vi "Comparator2.vi"(0 "7-have":i32, 1 "5-code":i32, 2 "6-have":i32, 3 "6-code":i32, 4 "5- have":i32, 5 "7-code":i32, 6 "8-code":i32, 8 "4-code":i32, 9 "1-have":i32, 10 "8-have":i32, 11 "2-have":i32, 12 "3 - code":i32, 13 "3- have":i32, 14 "2-code":i32, 15 "4-have":i32, 16 "1 - code":i32) -> (18 "Enough Marbles?":bool)   [LabVIEW 2016]
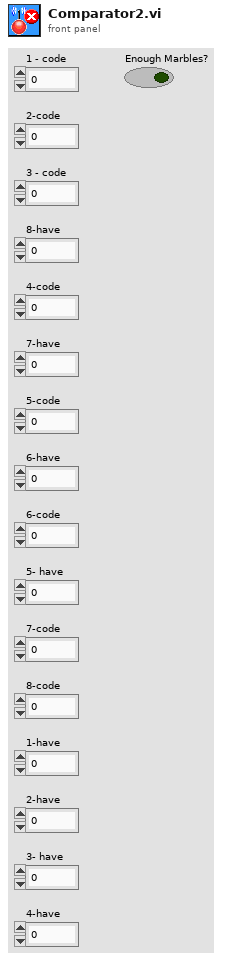
[diagram p1: front panel]
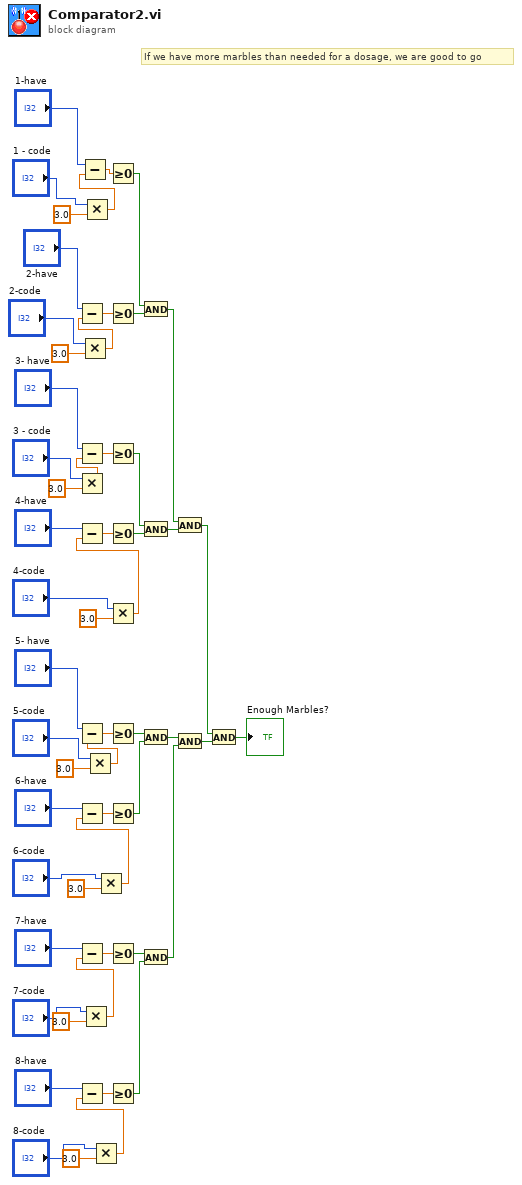
[diagram p0: block diagram]
diagram:
  # "If we have more marbles than needed for a dosage, we are good to go"
  n1 = Multiply(x="3 - code", y=3.0) -> (x*y=w17:dbl)
  n2 = Subtract(x="3- have", y=w17) -> (x-y=w35:dbl)
  n3 = Multiply(x="2-code", y=3.0) -> (x*y=w20:dbl)
  n4 = Subtract(x="2-have", y=w20) -> (x-y=w34:dbl)
  n5 = Multiply(x="7-code", y=3.0) -> (x*y=w4:dbl)
  n6 = Subtract(x="7-have", y=w4) -> (x-y=w39:dbl)
  n7 = Multiply(x="1 - code", y=3.0) -> (x*y=w23:dbl)
  n8 = Subtract(x="1-have", y=w23) -> (x-y=w33:dbl)
  n9 = Multiply(x="5-code", y=3.0) -> (x*y=w10:dbl)
  n10 = Subtract(x="5- have", y=w10) -> (x-y=w37:dbl)
  n11 = Multiply(x="8-code", y=3.0) -> (x*y=w1:dbl)
  n12 = Subtract(x="8-have", y=w1) -> (x-y=w40:dbl)
  n13 = Multiply(x="6-code", y=3.0) -> (x*y=w8:dbl)
  n14 = Subtract(x="6-have", y=w8) -> (x-y=w38:dbl)
  n15 = Greater Or Equal To 0?(x=w33) -> (x >= 0?=w41:bool)
  n16 = Greater Or Equal To 0?(x=w34) -> (x >= 0?=w42:bool)
  n17 = Greater Or Equal To 0?(x=w35) -> (x >= 0?=w43:bool)
  n18 = Multiply(x="4-code", y=3.0) -> (x*y=w13:dbl)
  n19 = Subtract(x="4-have", y=w13) -> (x-y=w36:dbl)
  n20 = Greater Or Equal To 0?(x=w36) -> (x >= 0?=w44:bool)
  n21 = Greater Or Equal To 0?(x=w37) -> (x >= 0?=w45:bool)
  n22 = Greater Or Equal To 0?(x=w38) -> (x >= 0?=w46:bool)
  n23 = Greater Or Equal To 0?(x=w39) -> (x >= 0?=w47:bool)
  n24 = Greater Or Equal To 0?(x=w40) -> (x >= 0?=w48:bool)
  n25 = And(x=w41, y=w42) -> (x .and. y?=w51:bool)
  n26 = And(x=w43, y=w44) -> (x .and. y?=w52:bool)
  n27 = And(x=w45, y=w46) -> (x .and. y?=w50:bool)
  n28 = And(x=w47, y=w48) -> (x .and. y?=w49:bool)
  n29 = And(x=w51, y=w52) -> (x .and. y?=w53:bool)
  n30 = And(x=w50, y=w49) -> (x .and. y?=w54:bool)
  n31 = And(x=w53, y=w54) -> (x .and. y?=→"Enough Marbles?":bool)
